vi "MTMount_getNextSample_AzimuthCableWrap.vi"(8 "error in (no error)":errorcluster, 11 "Azimuth_Cable_Wrap_Ctl":T1) -> (0 "error out":errorcluster, 2 "function return":i32, 3 "Azimuth_Cable_Wrap_Ctl out":T1)   [LabVIEW 2018, in "SALLV_MTMount.lvlib"]
doc: "int MTMount_shm_getNextSample_Azimuth_Cable_WrapLV(MTMount_Azimuth_Cable_WrapLV *Azimuth_Cable_Wrap_Ctl );"
uses:
  SALLV_MTMount.lvlib
  DataTypes/Azimuth_Cable_Wrap.ctl
  SALLV_MTMount.so
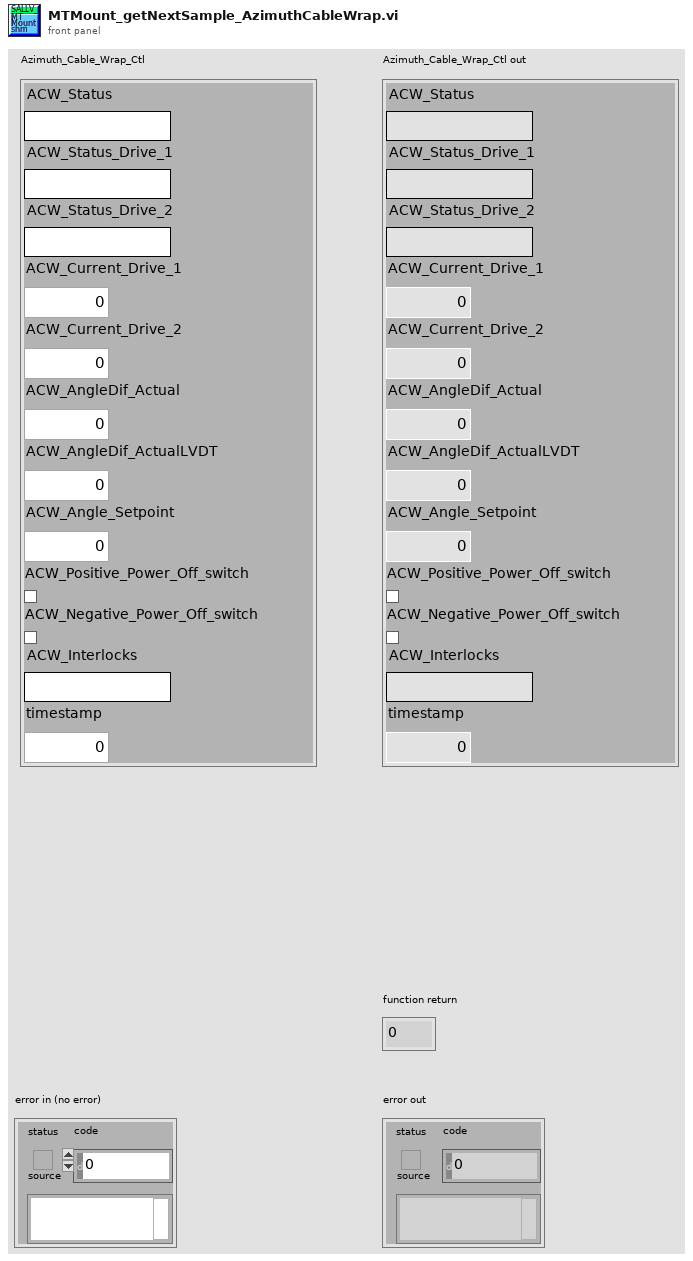
[diagram p1: front panel]
types:
  T1 = typedef "SALLV_MTMount.lvlib/Azimuth_Cable_Wrap.ctl" = cluster{"ACW_Status":string, "ACW_Status_Drive_1":string, "ACW_Status_Drive_2":string, "ACW_Current_Drive_1":dbl, "ACW_Current_Drive_2":dbl, "ACW_AngleDif_Actual":dbl, "ACW_AngleDif_ActualLVDT":dbl, "ACW_Angle_Setpoint":dbl, "ACW_Positive_Power_Off_switch":bool, "ACW_Negative_Power_Off_switch":bool, "ACW_Interlocks":string, "timestamp":dbl}
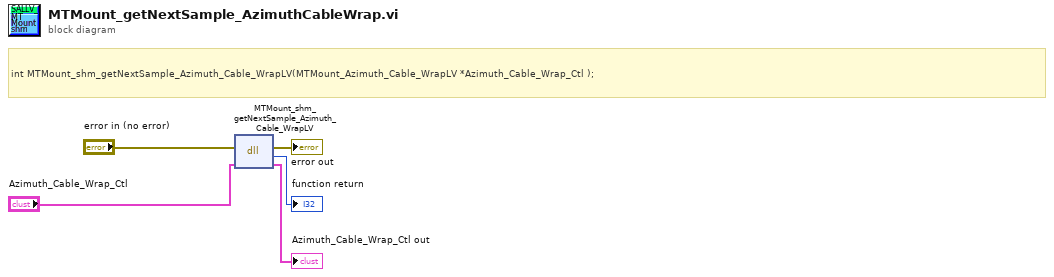
[diagram p0: block diagram]
diagram:
  # "int MTMount_shm_getNextSample_Azimuth_Cable_WrapLV(MTMount_Azimuth_Cable_WrapLV *Azimuth_Cable_Wrap_Ctl );"
  n1 = dll-call lib="home/ttsai/Document/salApiMTMount/SALLV_MTMount/SALLV_MTMount.*" fn="MTMount_shm_getNextSample_Azimuth_Cable_WrapLV"(error in="error in (no error)", "Azimuth_Cable_Wrap_Ctl"="Azimuth_Cable_Wrap_Ctl") -> (error out=→"error out":errorcluster, →"function return":i32, "Azimuth_Cable_Wrap_Ctl"=→"Azimuth_Cable_Wrap_Ctl out":T1)  [unwired: 2 in, 1 out]
